vi "Write From String Delimiter.vi"(8 "error in (no error)":errorcluster, 10 "Delimiter":string, 11 "Abs_Double Float 1D in":refnum<class "Abs_Single Float 1D.lvclass">) -> (0 "error out":errorcluster, 3 "Abs_Double Float 1D out":refnum<class "Abs_Single Float 1D.lvclass">)   [LabVIEW 2019, in "Abs_Single Float 1D.lvclass"]
uses:
  Abs_Single Float 1D.lvclass
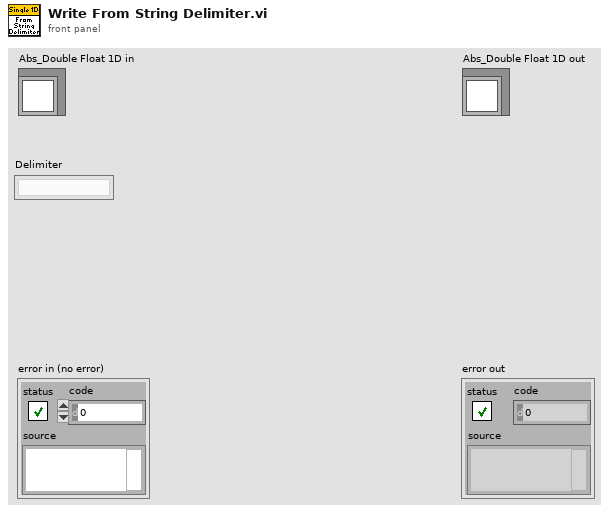
[diagram p1: front panel]
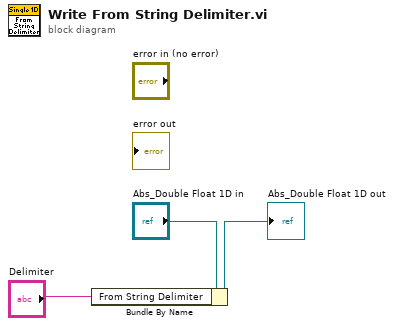
[diagram p0: block diagram]
diagram:
  n1 = Bundle By Name(cluster="Abs_Double Float 1D in", "From String Delimiter"="Delimiter") -> (→"Abs_Double Float 1D out":refnum<class "Abs_Single Float 1D.lvclass">)
